vi "Wavelet_Cluster_Database.vi"(0 "1-5 String Array Cluster":cluster{"1-5 String Array":string[]}={"1-5 String Array"=["1", "2", "3", "4", "5"]}, 1 "Orthogonal String Array Cluster":cluster{"Orthogonal String Array":string[]}={"Orthogonal String Array"=["1.1", "1.3", "1.5", "2.2", "2.4", "2.6", "2.8", "3.1", "3.3", "3.5", "3.7", "3.9", "4.4", "5.5", "6.8"]}, 2 "2-45 String Array Cluster":cluster{"2-45 String Array":string[]}={"2-45 String Array"=["2", "3", "4", "5", "6", "7", "8", "9", "10", "11", "12", "13", "14", "15", "16", "17", "18", "19", "20", "21", "22", "23", "24", "25", "26", "27", "28", "29", "30", "31", "32", "33", "34", "35", "36", "37", "38", "39", "40", "41", "42", "43", "44", "45"]}, 3 "Empty String Array Cluster":cluster{"Empty String Array":string[]}) -> ()   [LabVIEW 2014]
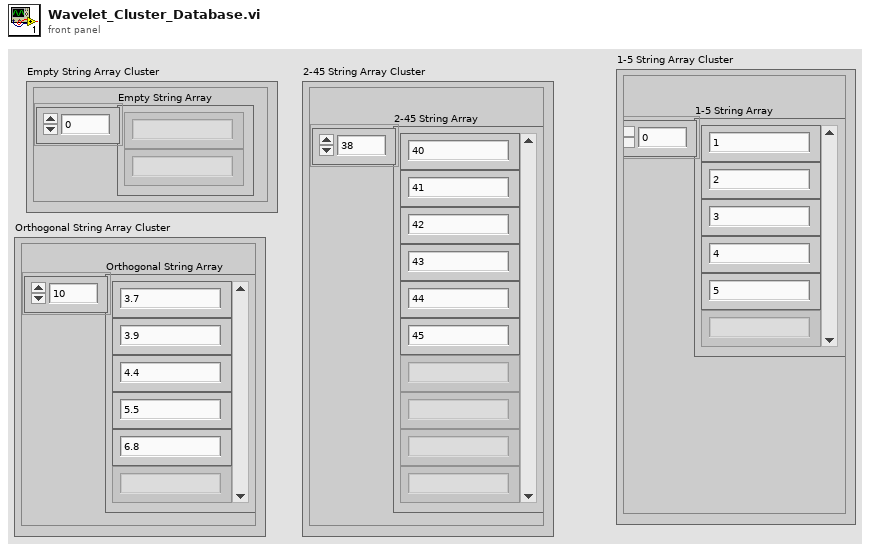
[diagram p1: front panel]
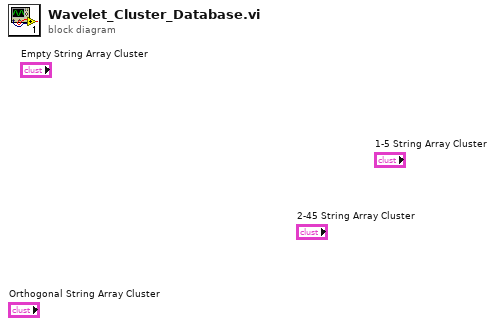
[diagram p0: block diagram]
diagram:
